vi "WPA.vi"(0 "System no.":i32=1 min=1 max=4 step=1, 2 "Affected axes":string[](array[string]), 3 "Password":string="100", 4 "Parameter no. format \n(Decimal: FALSE)":bool, 5 "error in":errorcluster, 6 "Parameter to save":i32[](array[numeric]), 7 "Parameter to save (hex)":u32[](array[numeric]) format="%.0x") -> (14 "Controller error":bool, 19 "error out":errorcluster)   [LabVIEW 2020]
doc: "If password is correct, this vi writes current settings of the given parameter numbers for Affected axes to non-volatile memory of the controller, waits 3000 ms (E-725, E-727: waits for controller ready by polling with #7) and queries ERR?. For axis-related parameters, Affected axes is the axis name, for piezo- or sensor-related parameters, the channel number, otherwise a parameter-related code. If parameter no. is in decimal format, use Parameter to save input, for hexadecimal parameter numbers use Parameter to save (hex) input and switch Parameter no. format to TRUE. Do not mix decimal and hex. parameter numbers in one call. See GCS DLL manual for available parameter numbers. If Affected axes is an empty array, WPA is sent without axis (item) and parameter specification.\n\nWARNING: \nIf current parameter values are incorrect, the system may malfunction. Be sure that you have the correct parameter settings before using the WPA command.\n\nC-413: Affected axes = empty array, the currently valid values of all parameters affected by the specified password are saved (see below). Parameter no. format is TRUE (hex). \nThe WPA command saves the currently valid parameter values to non-volatile memory, where they become the power-on defaults. Settings not saved with WPA will be lost when the C-413 is powered off or rebooted. Parameters can be changed in volatile memory with SPA, AOS, ATZ, CMO, RTR, VEL, WOS and WTR. Depending on the parameter to be saved, it may be necessary to switch to command level 1 (CCL.vi).\n\nC-867, C-877, C-891: Affected axes = empty array, the currently valid values of all parameters affected by the specified password are saved (see below). Parameter no. format is TRUE (hex). The WPA command saves the currently valid parameter values to non- volatile memory, where they become the power-on defaults. Settings not saved with WPA will be lost when the controller is powered off or rebooted. Parameters can be changed in volatile memory with SPA, ACC, DEC and VEL. WPA must be used without specifying any arguments except of the password, the currently valid values of all parameters affected by the specified password are saved.\n\nC-884: Affected axes = empty array, the currently valid values of all parameters affected by the specified password are saved (see below). Parameter no. format is TRUE (hex). Depending on the password, the WPA command saves the currently valid parameter values and/or the current HI device configuration to non-volatile memory, where they become the power-on defaults. Settings not saved with WPA will be lost when the controller is powered off or rebooted.\nValid passwords and affected settings:\n100: all parameters, settings of HDT, HIA, HIT \n101: all parameters \nHID: settings of HDT, HIA, HIT\nParameters can be changed in volatile memory with SPA, ACC, DEC and VEL.\nWPA must be used without specifying any arguments except of the password.\n\nC-886: See the user manual of the controller for valid passwords and affected settings.\n\nC-887, F-206, M-8X0: Check HLP?/HELP answer to find out if WPA is supported. Only for GCS syntax version = GCS 2.0 or higher (Check with CSV?.vi. IfCSV?.vi is not supported, syntax version is GCS 1.0). \nAffected axes and Parameter to save is only valid for Password = 100 or 101 (If Affected axes = empty array, all parameters for all axes are saved). Parameter no. format is TRUE (hex).\nDepending on the password, the WPA command saves the currently valid parameter values and/or the current coordinate systems settings or stage assignments to non-volatile memory, where they become the power-on defaults. Settings not saved with WPA will be lost when the controller is powered off or rebooted.\nValid passwords and affected settings:\nSKS: coordinate system settings A12: stage assignments for separate axes A and B 101: all parameters 100: all parameters and settings of SKS and A12 \nParameters can be changed in volatile memory with SPA.\n\nE-516: Affected axes and Parameter to save = empty array. E-516: The WPA command saves the currently valid parameters listed below to flash ROM, where they become the power-on defaults. Parameter changes not saved with WPA will be lost when the E-516 is powered off. Communication interface, enabled channels and display format, averaging (AVG), drift compensation mode (DCO), velocity control mode (VCO) and velocity (VEL), offset and gain for position and output voltage display, mode and tolerance for on-target reading (SPA), position limits (NLM, PLM), voltage limits (VMA, VMI), macros and default macro setting.\n\nE-517, E-518: If Affected axes = empty array, all parameters for all axes are saved. Parameter no. format is TRUE (hex). The WPA command saves the currently valid parameter values to non- volatile memory, where they become the power-on defaults. Settings not saved with WPA will be lost when the controller is powered off or rebooted. Parameters can be changed in volatile memory with SPA, IFC, SAI, DFH, VMI, VMA, WAV, WGC, WOS, WTR, RTR, and VEL. Furthermore, WPA saves the current settings of NLM, PLM (position soft limits), VCO (velocity control mode), DRC (data recorder configuration), CTO (trigger output configuration) and CSV (E-517 only. GCS syntax version, i.e. E-517 or E-516 mode; requires command level 1 (CCL.vi).\n\nE-709: If Affected axes = empty array, all parameters for all axes are saved. Parameter no. format is TRUE (hex). The WPA command saves the currently valid parameter values to non- volatile memory, where they become the power-on defaults. Settings not saved with WPA will be lost when the E-709 is powered off or rebooted. Parameters can be changed in volatile memory with SPA, AOS, ATZ, IFC, RTR, VEL, WOS and WTR. Depending on the parameter to be saved, it may be necessary to switch to command level 1 (CCL.vi).\n\nE-710: If Affected axes = empty array, all parameters for all axes are saved. See E-710 GCS DLL Manual for a list of available parameters. Command is available in command level 1 only (see CCL.vi and CCL?.vi). Parameter no. format is TRUE (hex.).\n\nE-712: If Affected axes = empty array, all parameters for all axes are saved. Parameter no. format is TRUE (hex). The WPA command saves the currently valid parameter values to non- volatile memory, where they become the power-on defaults. Settings not saved with WPA will be lost when the E-712 is powered off or rebooted. Parameters can be changed in volatile memory with SPA, AOS, ATZ, DPO, IFC, RTR, VEL, WOS and WTR. Requires command level 1 (CCL.vi). Do not save more than 10 parameters at once. \n\nE-725, E-727: The WPA command saves the currently valid parameter values to non- volatile memory, where they become the power-on defaults. Settings not saved with WPA will be lost when the E-725, E-727 is powered off or rebooted. Parameters can be changed in volatile memory with SPA, AOS, ATZ, DPO, IFC, RTR, VEL, WOS and WTR. Requires command level 1 (CCL.vi). As the WPA command takes up to 90 seconds to finish execution, WPA.vi polls for the controller ready signal (#7) before returning.\n\nE-753: If Affected axes = empty array, all parameters for all axes are saved. Parameter no. format is TRUE (hex). The WPA command saves the currently valid parameter values to non- volatile memory, where they become the power-on defaults. Settings not saved with WPA will be lost when the E-753 is powered off or rebooted. Parameters can be changed in volatile memory with SPA, AOS, ATZ, DPO, IFC, RTR, VEL, WOS and WTR. Requires command level 1 (CCL.vi).\n\nE-754: If Affected axes = empty array, all parameters for all axes are saved. Parameter no. format is TRUE (hex). The WPA command saves the currently valid parameter values to non- volatile memory, where they become the power-on defaults. Settings not saved with WPA will be lost when the E-754 is powered off or rebooted. Parameters can be changed in volatile memory with SPA, AOS, ATZ, DPO, IFC, RTR, VEL, WOS and WTR. \n\nE-755: If Affected axes = empty array, all parameters for all axes are saved. Parameter no. format is TRUE (hex). The WPA command saves the currently valid parameter values to non- volatile memory, where they become the power-on defaults. Settings not saved with WPA will be lost when the E-755 is powered off or rebooted. Parameters can be changed in volatile memory with SPA, APG, BDR and SSA. \n\nE-761: If Affected axes = empty array, all parameters for all axes (items) are saved. See E-7XX GCS DLL Manual for a list of available parameters. Parameter no. format is TRUE (hex.). The WPA command saves the currently valid parameter values and the additional settings listed below to non-volatile memory, where they become the power-on defaults. Settings not saved with WPA will be lost when the PC is powered off or the E-761 is rebooted. Additonal settings saved with WPA: Velocity control mode (VCO), position limits (NLM, PLM).\n\nE-816: Affected axes and Parameter to save = empty array. This command cannot be issued to a slave.\n\nE-861: The WPA command saves the currently valid parameter values to non- volatile memory, where they become the power-on defaults. Settings not saved with WPA will be lost when the E-861 is powered off or rebooted.\nThe password for writing to non-volatile memory depends on the parameter and can be \"100\" or \"4711\". See the parameter list in \"Controller Parameters\" in the E-861 user manual for the password assignment.\nWhen WPA is used without specifying any arguments except of the password, the currently valid values of all parameters affected by the specified password are saved. Otherwise only one single parameter can be saved per WPA command. Parameters can be changed in volatile memory with SPA, SSA, ACC, DEC, VEL, OVL, OAC and ODC. If Affected axes = empty array, the currently valid values of all parameters affected by the specified password are saved (see below). Parameter no. format is TRUE (hex).\n\nE-870, E-872: If Affected axes = empty array, all parameters for all axes are saved. Parameter no. format is TRUE (hex). The WPA command saves the currently valid parameter values to non- volatile memory, including the joystick configuration, where they become the power-on defaults. Settings not saved with WPA will be lost when the controller is powered off or rebooted. Parameters can be changed in volatile memory with SPA. \n\nE-871, E-873: If Affected axes = empty array, all parameters for all axes are saved. Parameter no. format is TRUE (hex). Depending on the password, the WPA command saves the currently valid parameter values and/or the current HI device configuration to non-volatile memory, where they become the power-on defaults. Settings not saved with WPA will be lost when the controller is powered off or rebooted.\nValid passwords and affected settings:\n100: all parameters, settings of HDT, HIA, HIT \n101: all parameters \nHID: settings of HDT, HIA, HIT\nParameters can be changed in volatile memory with SPA.\nWPA must be used without specifying any arguments except of the password.\n\nE-874: If Affected axes = empty array, all parameters for all axes are saved. Parameter no. format is TRUE (hex). Depending on the password, the WPA command saves the currently valid parameter values and/or the current HI device configuration to non-volatile memory, where they become the power-on defaults. Settings not saved with WPA will be lost when the controller is switched off or rebooted.\nValid passwords and affected settings:\n100: all parameters\nParameters can be changed in volatile memory with SPA.\nWPA must be used without specifying any arguments except of the password.\n\nHydra, Pollux: Affected axes = empty array, the currently valid values of all parameters affected by the specified password are saved (see below). Parameter no. format is TRUE (hex). The WPA command saves the currently valid parameter values to non-volatile memory, where they become the power-on defaults. Settings not saved with WPA will be lost when the controller is powered off or rebooted. Parameters can be changed in volatile memory with SPA, ACC, and VEL. WPA must be used without specifying any arguments except of the password, the currently valid values of all parameters affected by the specified password are saved.\n\nMercury_GCS: Affected axes = empty array, the currently valid values of all parameters affected by the specified password are saved (see below). Parameter no. format is TRUE (hex). The WPA command saves the currently valid parameter values to non-volatile memory, where they become the power-on defaults. Settings not saved with WPA will be lost when the Mercury is powered off or rebooted. Parameters can be changed in volatile memory with SPA, ACC, DEC and VEL.WPA must be used without specifying any arguments except of the password, the currently valid values of all parameters affected by the specified password are saved."
uses:
  General command.llb/Controller names.ctl
  General command.llb/Global2 (Array).vi
panel:
  in  "Local stop":bool
  in  "Stop refnum":refnum<vi>
  # "If password is correct, this vi writes current settings of the given parameter numbers  for \"Affected axes\" to  non-volatile memory\nof the controller, waits 3000 ms (E-725: waits for controller ready by polling with #7) and queries ERR?.  If parameter no. is in decimal\nformat, use \"Parameter to save\" input, for hexadecimal parameter numbers use \"Parameter to save (hex)\" input and switch \n\"Parameter no. format\" to TRUE.  Do not mix decimal and hex. parameter numbers in one call. See GCS DLL manual for available \nparameter numbers. If \"Affected axes\" is an empty array, WPA is sent without axis and parameter specification."
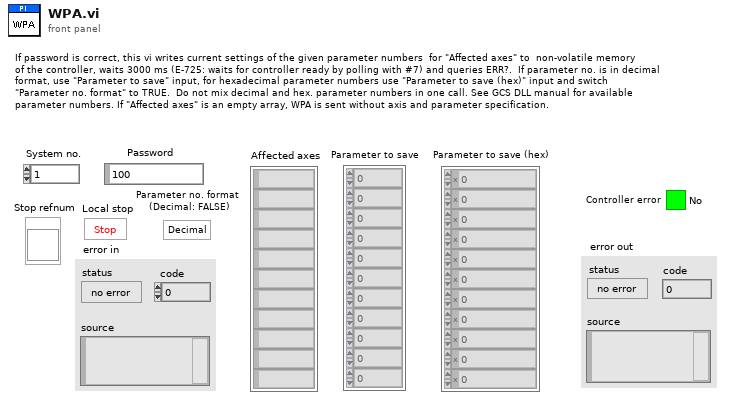
[diagram p1: front panel]
types:
  T1 = typedef "Controller names.ctl" = enum16{"None", "Analog", "C-702", "C-413", "C-414", "C-843", "C-843.PM", "C-844", "C-848", "C-865", "C-866", "C-867", "C-877", "C-880", "C-884", "C-885", "C-886", "C-887", "C-891", "E-135", "E-516", "E-517", "E-518", "E-709", "E-710", "E-712", "E-725", "E-727", "E-753", "E-754", "E-755", "E-761", "E-816", "E-861", "E-870", "E-871", "E-872", "E-873", "E-874", "F-206", "HydraPollux", "M-840", "M-850", "M-8X0", "Mercury", "Mercury_GCS", "PI_GCS2"}
  T2 = cluster{"Conn. axes":string[], "Controller name":T1}[]
  T3 = cluster{"Conn. axes":string[], "Controller name":T1}
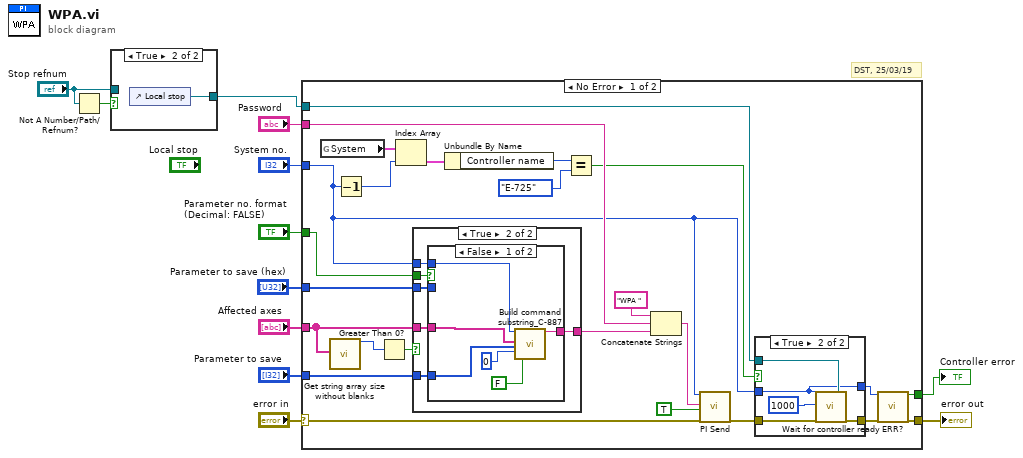
[diagram p0: block diagram]
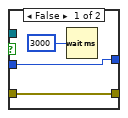
[diagram p3: hidden frame]
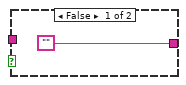
[diagram p4: hidden frame]
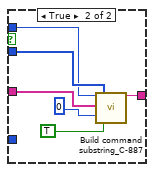
[diagram p5: hidden frame]
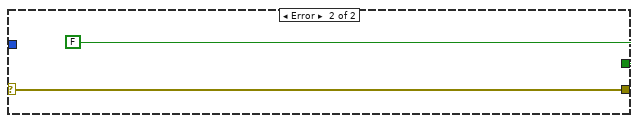
[diagram p6: hidden frame]
diagram:
  # "DST, 25/03/19"
  n1 = Not A Number/Path/Refnum?(number/path/refnum="Stop refnum") -> (NaN/Path/Refnum?=w4:bool)
  n2 = case shown="True" w4 {
    tunnel: [w13 w14] -> w2
    tunnel: "Stop refnum" -> [w13 _]
    frame False {
    }
    frame True {
      n3 = control-ref of="Local stop"() -> (w14:refnum<vi>)
    }
  }
  n4 = case shown="No Error" "error in" {
    selector: "error in" -> [w21 w67]
    tunnel: [w39 w67] -> w12
    tunnel: "System no." -> [w19 _]
    tunnel: "Password" -> [w36 _]
    tunnel: [w35 FALSE ("Controller error")] -> w10
    tunnel: "Affected axes" -> [w31 _]
    tunnel: "Parameter to save" -> [w32 _]
    tunnel: "Parameter to save (hex)" -> [w27 _]
    tunnel: "Parameter no. format \n(Decimal: FALSE)" -> [w26 _]
    tunnel: w2 -> [w22 _]
    frame No Error {
      n5 = global read "Global2 (Array).vi" "System"() -> (w20:T2)
      n6 = call "Get string array size without blanks.vi"("String array"=w31) -> ("Corrected array size"=w30:i32)  [unwired: 18 out]
      n7 = Decrement(x=w19) -> (x-1=w18:i32)
      n8 = Greater Than 0?(x=w30) -> (x > 0?=w29:bool)
      n9 = Index Array(array=w20, index=w18) -> (element=w17:T3)
      n10 = case shown="True" w29 {
        tunnel: w31 -> [_ w54]
        tunnel: w32 -> [_ w53]
        tunnel: ["" ("Command substring") w52] -> w28
        tunnel: w27 -> [_ w50]
        tunnel: w26 -> [_ w51]
        tunnel: w19 -> [_ w49]
        frame False {
        }
        frame True {
          n11 = case shown="False" w51 {
            tunnel: w54 -> [w59 w65]
            tunnel: w53 -> [w58 _]
            tunnel: [w57 w64] -> w52
            tunnel: w50 -> [_ w62]
            tunnel: w49 -> [w55 w61]
            frame False {
              n12 = call "Build command substring_C-887.vi"("System no."=w55, "Affected axes"=w59, "Parameters"=w58, "No. of digits"=i16 0, "Parameter no. format \n(Decimal: FALSE)"=FALSE ("Parameter no. format \n(Decimal: FALSE)")) -> ("Command substring"=w57:string)  [unwired: 2 in, 12 out]
            }
            frame True {
              n13 = call "Build command substring_C-887.vi"("System no."=w61, "Affected axes"=w65, "No. of digits"=i16 0, "Parameters (hex)"=w62, "Parameter no. format \n(Decimal: FALSE)"=TRUE ("Parameter no. format \n(Decimal: FALSE)")) -> ("Command substring"=w64:string)  [unwired: 2 in, 12 out]
            }
          }
        }
      }
      n14 = Unbundle By Name(w17) -> ("Controller name"=w25:T1)
      n15 = Equal?(x=w25, y=Controller_names."E-725") -> (x = y?=w23:bool)
      n16 = Concatenate Strings("WPA ", w36, w28) -> (w37:string)
      n17 = call "PI Send.vi"("System no."=w19, "String to send"=w37, "Attach termination char.?"=TRUE ("Attach Linefeed?"), "error in"=w21) -> ("error out"=w34:errorcluster)  [unwired: 2 in, 13 out]
      n18 = case shown="True" w23 {
        tunnel: w34 -> [w41 w47]
        tunnel: [w41 w46] -> w33
        tunnel: w19 -> [w40 w43]
        tunnel: w22 -> [_ w45]
        tunnel: [w40 w43] -> w15
        frame False {
          n19 = Wait (ms)(milliseconds to wait=u32 3000 ("millisecond timer value")) -> ()  [unwired: 1 out]
        }
        frame True {
          n20 = call "Wait for controller ready.vi"("System no."=w43, "Polling time, ms"=1000, "error in"=w47, "Stop refnum"=w45) -> ("error out"=w46:errorcluster)  [unwired: 15 out]
        }
      }
      n21 = call "ERR?.vi"("System no."=w15, "error in"=w33) -> ("Controller error"=w35:bool, "error out"=w39:errorcluster)  [unwired: 16 out]
    }
    frame Error {
    }
  }
  "error out" <- w12
  "Controller error" <- w10
